vi "S2C_ExeScriptExecute.vi"(8 "Error In":errorcluster, 11 "Q-Ref":refnum<queue>) -> (0 "Error Out":errorcluster)   [LabVIEW 2015]
doc: "Executes the actions associated with a line item and updates the results cell in the execution table."
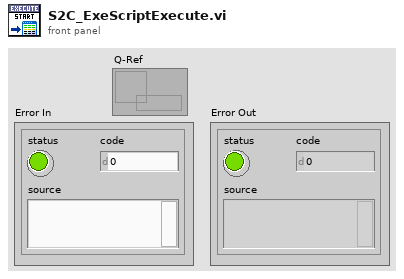
[diagram p1: front panel]
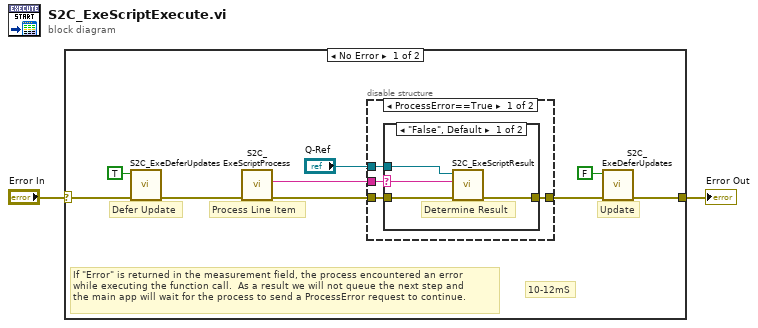
[diagram p0: block diagram]
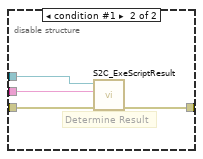
[diagram p3: hidden frame]
diagram:
  n1 = case shown="No Error" "Error In" {
    selector: "Error In" -> [w3 w25]
    tunnel: [w4 w25] -> w1
    frame No Error {
      # "Update"
      # "Defer Update"
      # "10-12mS"
      # "If \"Error\" is returned in the measurement field, the process encountered an error\nwhile executing the function call.  As a result we will not queue the next step and\nthe main app will wait for the process to send a ProcessError request to continue."
      # "Process Line Item"
      n2 = call "S2C_ExeDeferUpdates.vi"("Error In"=w3, "Defer?"=TRUE) -> ("Error Out"=w8:errorcluster)  [unwired: 9 in]
      n3 = call "S2C_ExeScriptProcess.vi"("Error In"=w8) -> ("Error Out"=w9:errorcluster, "Measurement"=w10:string)  [unwired: 9 in]
      n4 = disable-structure shown="ProcessError==True" {
        disable-tunnel: w9 -> [w15 w24]
        disable-tunnel: [w14 w23] -> w5
        disable-tunnel: "Q-Ref" -> [w12 w22]
        disable-tunnel: w10 -> [w13 w21]
        frame condition #0 (active) {
          n5 = case shown="\"False\", Default" w13 {
            selector: w13 -> [w16 _]
            tunnel: w15 -> [w19 w20]
            tunnel: [w18 w20] -> w14
            tunnel: w12 -> [w17 _]
            frame "False", Default {
              # "Determine Result"
              n6 = call "S2C_ExeScriptResult.vi"("Error In"=w19, "Measurement"=w16, "Q_Ref"=w17) -> ("Error Out"=w18:errorcluster)  [unwired: 8 in]
            }
            frame "Error" {
            }
          }
        }
        frame condition #1 {
          # "Determine Result"
          n7 = call "S2C_ExeScriptResult.vi"("Error In"=w24, "Measurement"=w21, "Q_Ref"=w22) -> ("Error Out"=w23:errorcluster)  [unwired: 8 in]
        }
      }
      n8 = call "S2C_ExeDeferUpdates.vi"("Error In"=w5, "Defer?"=FALSE) -> ("Error Out"=w4:errorcluster)  [unwired: 9 in]
    }
    frame Error {
    }
  }
  "Error Out" <- w1
